vi "DFD Integer Delay with State (PtByPt).vi"(6 "state in":dbl[](array[numeric]), 8 "error in (no error)":errorcluster, 10 "delay":i32=1, 11 "signal in":dbl) -> (0 "error out":errorcluster, 3 "signal out":dbl, 4 "state out":dbl[](array[numeric]))   [LabVIEW 2017, in "NI_DigFilterLicensed.lvlib"]
doc: "Delays a signal by a specified integer number of sample intervals. You must specify the initial internal states in the <B>state in</B> input to generate an accurate output. Wire data to the <B>signal in</B> input to determine the polymorphic instance to use or manually select the instance."
uses:
  <vilib>/addons/Digital Filter Design/NI_DigFilterLicensed.lvlib
  <vilib>/addons/Digital Filter Design/NI_DigFilter_Process.lvlib
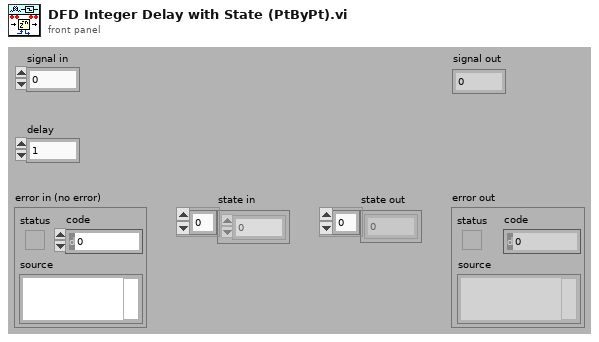
[diagram p1: front panel]
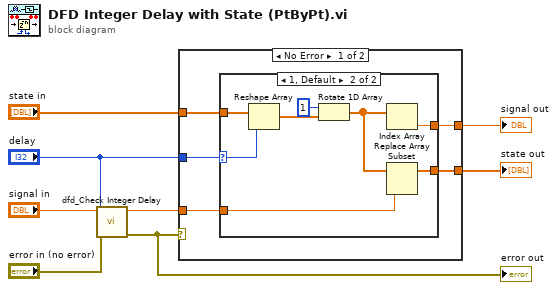
[diagram p0: block diagram]
diagram:
  n1 = call <vilib>:"dfd_Check Integer Delay.vi"("error in (no error)"="error in (no error)", "delay in"="delay") -> ("error out"=w5:errorcluster)  [unwired: 9 out]
  "error out" <- w5
  n2 = case shown="No Error" w5 {
    tunnel: "state in" -> [w12 _]
    tunnel: "delay" -> [w8 _]
    tunnel: [w9 _] -> w6
    tunnel: "signal in" -> [w10 _]
    tunnel: [w11 _] -> w1
    frame No Error {
      n3 = case shown="1, Default" w8 {
        selector: w8 -> [_ w14]
        tunnel: w12 -> [_ w21]
        tunnel: [w13 w19] -> w11
        tunnel: w10 -> [w13 w17]
        tunnel: [_ w16] -> w9
        frame 0 {
        }
        frame 1, Default {
          n4 = Reshape Array(w21, w14) -> (w15:dbl[])
          n5 = Rotate 1D Array(1:w15, 2:1 ("n")) -> (0:w18:dbl[])
          n6 = Index Array(array=w18) -> (element=w19:dbl)  [unwired: 1 in]
          n7 = Replace Array Subset(array=w18, new element=w17) -> (w16:dbl[])  [unwired: 1 in]
        }
      }
    }
    frame Error {
    }
  }
  "signal out" <- w1
  "state out" <- w6
